vi "disk_appendTimeFormat.vi"(7 "columns":T5, 8 "error in (no error)":errorcluster, 11 "DiskTemplate":T1={"XMLRef"=[refnum, refnum, refnum, refnum, refnum, refnum], "ZipPath"=path "", "MetaFile"={"Ref"=refnum, "NextRow"=0, "NextPosition"=0, "Block"=[]}, "TempFolder"=path ""}) -> (0 "error out":errorcluster, 1 "styles map":string[](array[string]), 2 "max existed styles":i32, 3 "DiskTemplate out":T1)   [LabVIEW 2017, in "NI_ExcelFile.lvlib"]
uses:
  <vilib>/express/express shared/NI_ExcelFile/NI_ExcelFile.lvlib
  <vilib>/express/express shared/NI_ExcelFile/Ctrls/disk_TemplateFile.ctl
  <vilib>/express/express shared/NI_ExcelFile/Ctrls/meta_file.ctl
  <vilib>/express/express shared/NI_ExcelFile/Ctrls/meta_Block.ctl
  <vilib>/express/express shared/NI_ExcelFile/Ctrls/meta_BlockType.ctl
  <vilib>/express/express shared/NI_ExcelFile/Ctrls/Columns.ctl
  <vilib>/express/express shared/NI_ExcelFile/Ctrls/ColumnInfo.ctl
  <vilib>/express/express shared/NI_ExcelFile/Ctrls/DataType.ctl
  <vilib>/express/express shared/NI_ExcelFile/Ctrls/TemplateEnum.ctl
  <vilib>/express/express shared/NI_ExcelFile/Ctrls/meta_ColumnInfo_2013.ctl
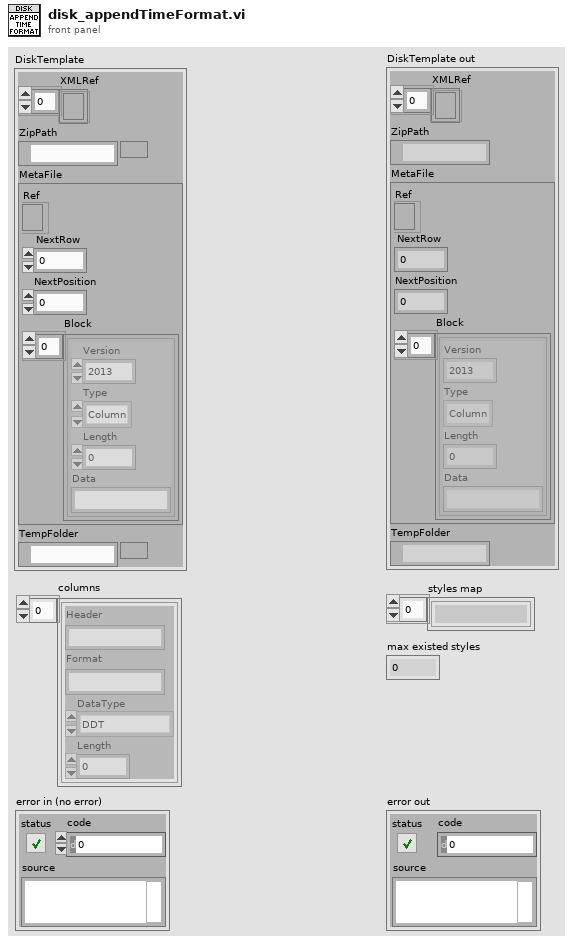
[diagram p1: front panel]
types:
  T1 = typedef "NI_ExcelFile.lvlib/disk_TemplateFile.ctl" = cluster{"XMLRef":refnum<file>[], "ZipPath":path, "MetaFile":T2, "TempFolder":path}
  T2 = typedef "NI_ExcelFile.lvlib/meta_file.ctl" = cluster{"Ref":refnum<file>, "NextRow":i32, "NextPosition":i64, "Block":T3[]}
  T3 = typedef "NI_ExcelFile.lvlib/meta_Block.ctl" = cluster{"Version":u16, "Type":T4, "Length":i32, "Data":string}
  T4 = typedef "NI_ExcelFile.lvlib/meta_BlockType.ctl" = enum16{"NITag", "File", "Column"}
  T5 = typedef "NI_ExcelFile.lvlib/Columns.ctl" = T6[]
  T6 = typedef "NI_ExcelFile.lvlib/ColumnInfo.ctl" = cluster{"Header":string, "Format":string, "DataType":T7, "Length":u64}
  T7 = typedef "NI_ExcelFile.lvlib/DataType.ctl" = enum16{"DDT", "WFM", "Array of STR", "Array of DBL", "Array of I8", "Array of I16", "Array of I32", "Array of I64", "Array of SGL", "Array of U8", "Array of U16", "Array of U32", "Array of U64", "Array of Time"}
  T8 = typedef "NI_ExcelFile.lvlib/meta_ColumnInfo_2013.ctl" = cluster{"Index":i32, "DataType":T7, "Header":string, "Format":string, "StartRow":i32, "Length":i32}
  T9 = typedef "NI_ExcelFile.lvlib/TemplateEnum.ctl" = enum16{"[Content_Types].xml", ".rels", "workbook.xml", "styles.xml", "workbook.xml.rels", "sheet.xml", "app.xml", "core.xml"}
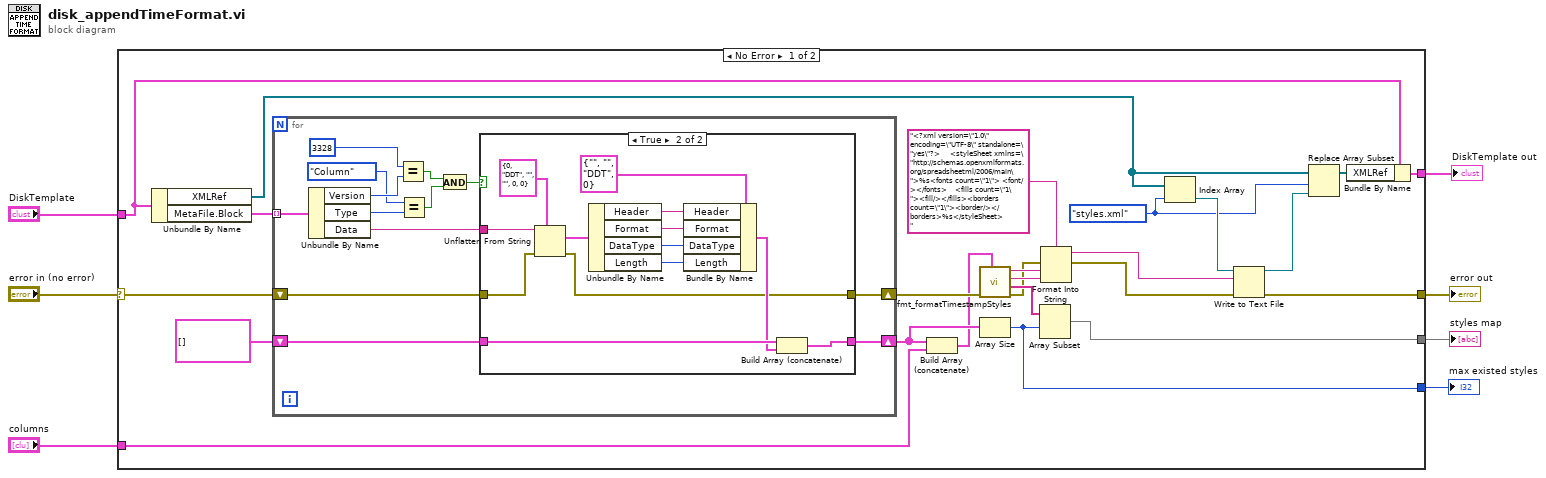
[diagram p0: block diagram]
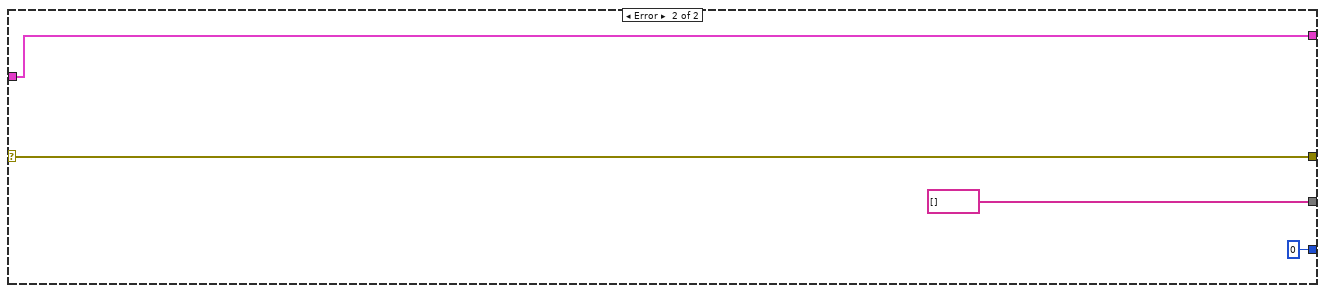
[diagram p3: hidden frame]
diagram:
  n1 = case shown="No Error" "error in (no error)" {
    selector: "error in (no error)" -> [w29 w62]
    tunnel: "DiskTemplate" -> [w17 w61]
    tunnel: "columns" -> [w27 _]
    tunnel: [w24 string[] []] -> w4
    tunnel: [w23 w62] -> w3
    tunnel: [w18 w61] -> w2
    tunnel: [w8 0] -> w1
    frame No Error {
      w19 = TemplateEnum."styles.xml" ("Template")
      n2 = Unbundle By Name(w17) -> ("XMLRef"=w21:refnum<file>[], "MetaFile.Block"=w31:T3[])
      n3 = for {
        tunnel: w31 -> [w44] mode=indexing
        shift-right: [w34] -> w26
        shift-left: T5 [] ("Columns") -> [w35]
        shift-right: [w33] -> w28
        shift-left: w29 -> [w32]
        n4 = Unbundle By Name(w44) -> ("Version"=w39:u16, "Type"=w40:T4, "Data"=w36:string)
        n5 = Equal?(x=u16 3328 ("Version"), y=w39) -> (x = y?=w42:bool)
        n6 = Equal?(x=meta_BlockType."Column" ("Type"), y=w40) -> (x = y?=w41:bool)
        n7 = And(x=w42, y=w41) -> (x .and. y?=w43:bool)
        n8 = case shown="True" w43 {
          tunnel: w36 -> [_ w59]
          tunnel: w35 -> [w46 w57]
          tunnel: [w46 w56] -> w34
          tunnel: [w45 w48] -> w33
          tunnel: w32 -> [w45 w47]
          frame False {
          }
          frame True {
            n9 = Unflatten From String(type=T8 {"Index"=0, "DataType"=enum."DDT", "Header"="", "Format"="", "StartRow"=0, "Length"=0} ("meta_ColumnInfo_2013"), binary string=w59, error in (no error)=w47) -> (value=w53:T8, error out=w48:errorcluster)  [unwired: 2 in, 1 out]
            n10 = Unbundle By Name(w53) -> ("Header"=w52:string, "Format"=w51:string, "DataType"=w50:T7, "Length"=w49:i32)
            n11 = Bundle By Name(cluster=T6 {"Header"="", "Format"="", "DataType"=enum."DDT", "Length"=0} ("Column"), "Header"=w52, "Format"=w51, "DataType"=w50, "Length"=w49) -> (w54:T6)
            n12 = Build Array (concatenate)(w57, w54) -> (w56:T5)
          }
        }
      }
      n13 = Build Array (concatenate)(w26, w27) -> (w9:T5)
      n14 = call <vilib>:"fmt_formatTimestampStyles.vi"("Columns"=w9, "error in"=w28) -> ("error out"=w12:errorcluster, "styles map"=w25:string[], "cellXfs"=w14:string, "numFmts"=w15:string)  [unwired: 6 in]
      n15 = Array Size(array=w26) -> (size(s)=w8:i32)
      n16 = Array Subset(array=w25, index=w8) -> (w24:string[])  [unwired: 1 in]
      n17 = Format Into String(format string="<?xml version=\"1.0\" encoding=\"UTF-8\" standalone=\"yes\"?>     <styleSheet xmlns=\"http://schemas.openxmlformats.org/spreadsheetml/2006/main\">%s<fonts count=\"1\"> <font/></fonts>    <fills count=\"1\"><fill/></fills><borders count=\"1\"><border/></borders>%s</styleSheet>              " ("string"), error in=w12, w15, w14) -> (resulting string=w13:string, error out=w11:errorcluster)  [unwired: 1 in]
      n18 = Index Array(array=w21, index=w19) -> (element=w22:refnum<file>)
      n19 = Write to Text File(file (use dialog)=w22, text=w13, error in=w11) -> (refnum out=w20:refnum<file>, error out=w23:errorcluster)  [unwired: 1 in, 1 out]
      n20 = Replace Array Subset(array=w21, new element=w20, index=w19) -> (w16:refnum<file>[])
      n21 = Bundle By Name(cluster=w17, "XMLRef"=w16) -> (w18:T1)
    }
    frame Error {
    }
  }
  "error out" <- w3
  "styles map" <- w4
  "DiskTemplate out" <- w2
  "max existed styles" <- w1
